vi "Funcionamiento_listbox.vi"() -> ()   [LabVIEW 2019]
panel:
  in  "Invent":dbl
  in  "Multicolumn Listbox":i32(listbox)
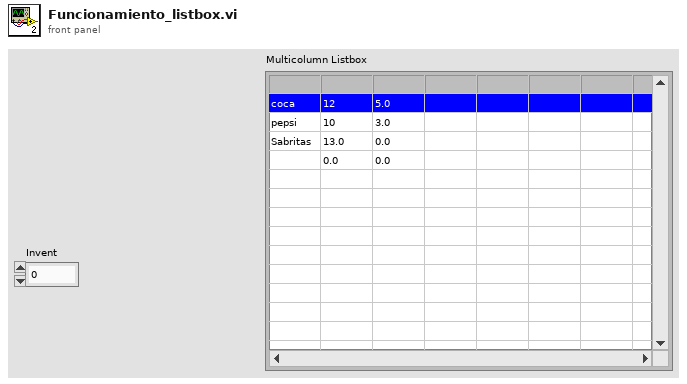
[diagram p1: front panel]
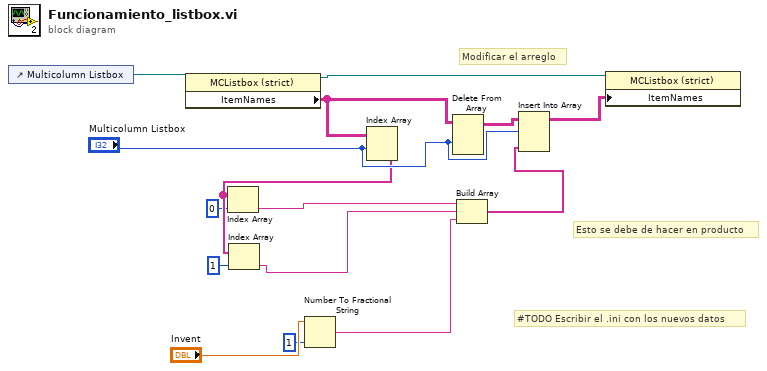
[diagram p0: block diagram]
diagram:
  # "Esto se debe de hacer en producto"
  # "#TODO Escribir el .ini con los nuevos datos"
  # "Modificar el arreglo"
  n1 = control-ref of="Multicolumn Listbox"() -> (w15:refnum<vi>)
  n2 = property class="MCListbox (strict)"(reference=w15) -> (reference out=w7:refnum<vi>, "ItemNames"=w11:string[][])  [unwired: 1 in, 1 out]
  n3 = Number To Fractional String(number="Invent", precision (6)=i16 1) -> (F-format string=w12:string)  [unwired: 2 in]
  n4 = Index Array(array=w11, index (row)="Multicolumn Listbox") -> (element=w5:string[])  [unwired: 1 in]
  n5 = Index Array(array=w5, index=0) -> (element=w1:string)
  n6 = Index Array(array=w5, index=1) -> (element=w2:string)
  n7 = Delete From Array(array=w11, index (row)="Multicolumn Listbox") -> (array with subset deleted=w6:string[][])  [unwired: 2 in, 1 out]
  n8 = Build Array(w1, w2, w12) -> (w9:string[])
  n9 = Insert Into Array(array=w6, index (row)="Multicolumn Listbox", new element=w9) -> (w8:string[][])  [unwired: 1 in]
  n10 = property class="MCListbox (strict)"(reference=w7, "ItemNames"=w8) -> ()  [unwired: 1 in, 2 out]
